vi "GB Test for MANU.vi"(8 "error in":errorcluster, 11 "VISA resource name":refnum<visa-resource-name>) -> (0 "error out":errorcluster, 3 "VISA resource name out":refnum<visa-resource-name>)   [LabVIEW 2011, in "GPT-9000.lvlib"]
uses:
  <instrlib>/GPT-9000/GPT-9000.lvlib
panel:
  in  "GB reference value(m£[)":sgl min=0 max=649.9 format="%.1f"
  in  "GB Test Frequency(Hz)":u8(ring)=1 items=["50", "60"]
  in  "GB Test Time(S)":sgl=2.0 min=0.5 max=999.9 format="%.1f"
  in  "GB LO SET resistance value(m£[)":sgl=0.1 min=0.1 max=649.9 format="%.1f"
  in  "GB HI SET resistance value(m£[)":sgl=650.0 min=0.1 max=650 format="%.1f"
  in  "GB current(A)":sgl=3.0 min=3 max=32 format="%.2f"
  in  "Clear Error(True)":bool=TRUE
  in  "ID Query (True)":bool=TRUE
  out "ID Return String":string
  in  "Start":bool
  in  "Stop":bool
  in  "Test number":u8 max=100
  out "Error Message":string
  out "Error LED":bool
  in  "Test name":string="TEST_NAME"
  out "Time":string
  out "Current":string
  out "Impedance":string
  out "READY":bool
  out "TEST":bool
  out "PASS":bool
  out "FAIL":bool
  out "LED":bool
  out "Ready to Start":bool
  in  "Configure RS232 Baud Rate":u32(ring)=115200 items=["9600"=9600, "19200"=19200, "38400"=38400, "57600"=57600, "115200"=115200]
  # "GB Test for MANU Mode"
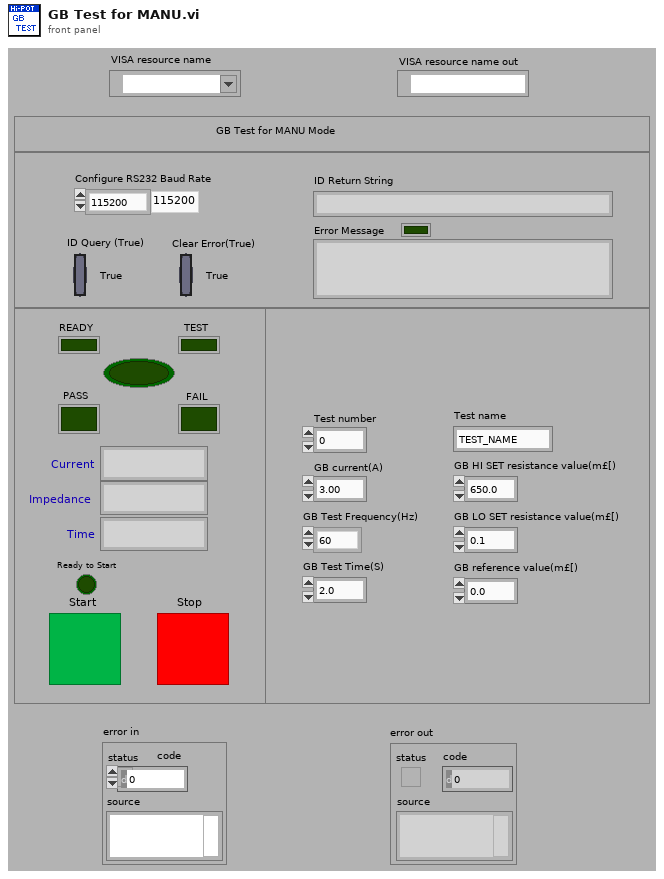
[diagram p1: front panel]
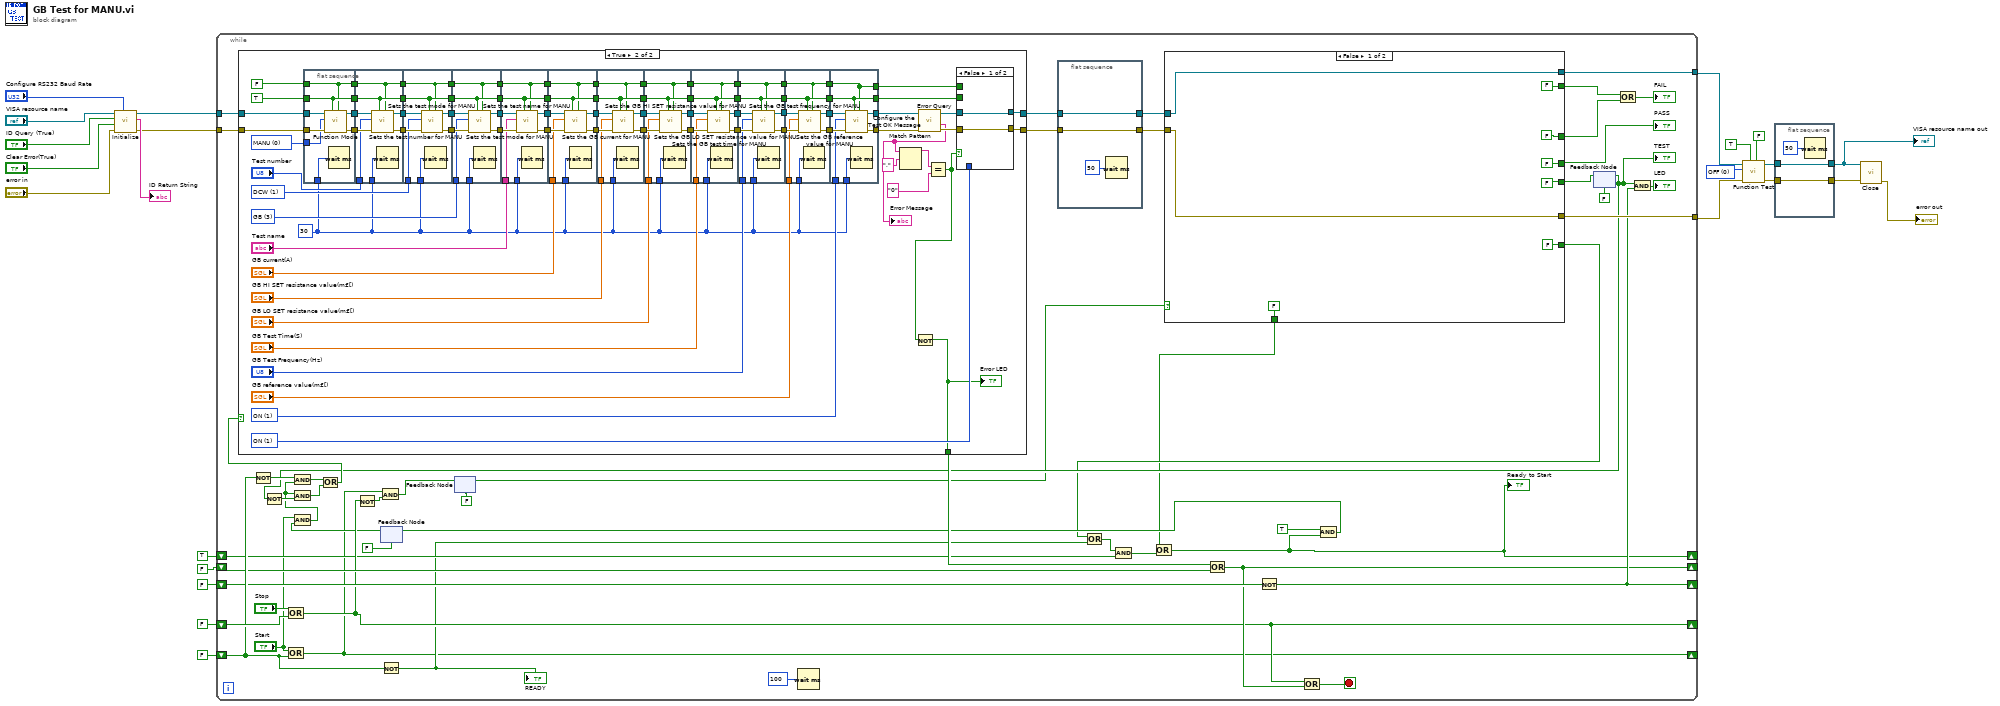
[diagram p0: block diagram]
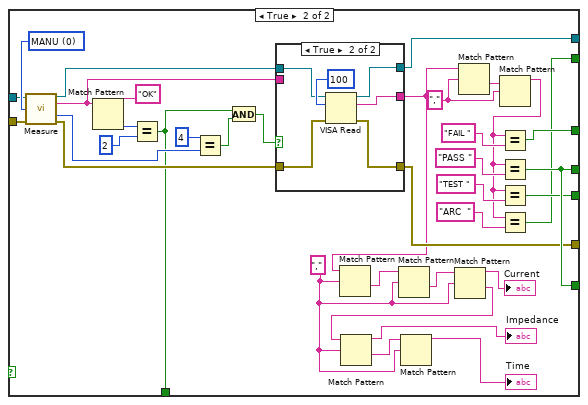
[diagram p2: hidden frame]
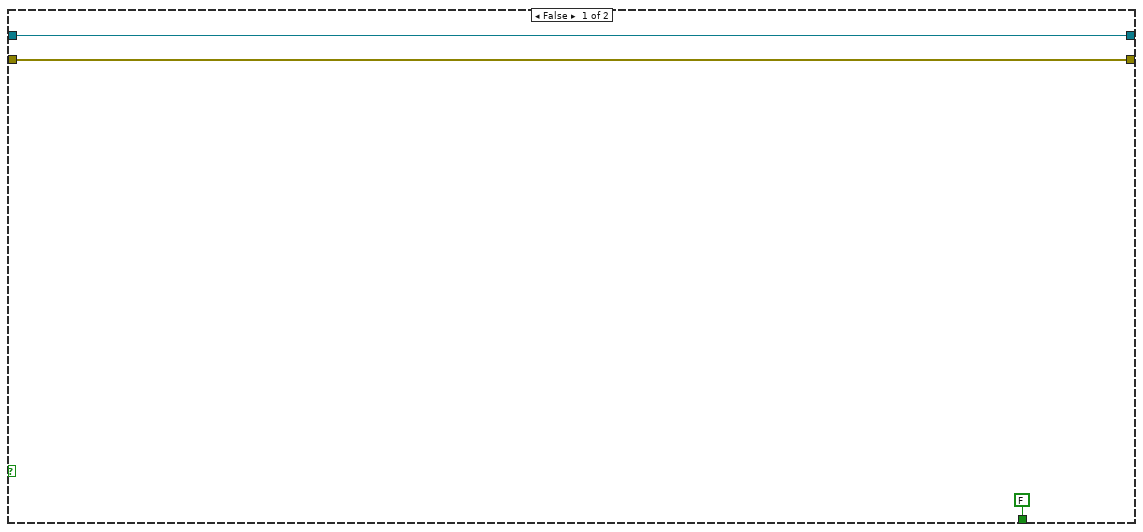
[diagram p4: hidden frame]
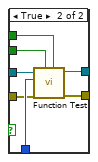
[diagram p5: hidden frame]
diagram:
  w21 = u8 0 items=["OFF", "ON"] ("Function Test")
  n1 = call <instrlib>:"Initialize.vi"("Configure RS232 Baud Rate"="Configure RS232 Baud Rate", "error in (no error)"="error in", "Clear Error(True)"="Clear Error(True)", "ID Query (True)"="ID Query (True)", "VISA resource name"="VISA resource name") -> ("error out"=w10:errorcluster, "ID Return String"=→"ID Return String":string, "VISA resource name out"=w11:refnum<visa-resource-name>)  [unwired: 3 in, 1 out]
  n2 = while {
    shift-right: [w30] -> _
    shift-left: FALSE -> [w66]
    shift-right: [w51] -> _
    shift-left: FALSE -> [w72]
    tunnel: [w71] -> w23
    tunnel: [w70] -> w22
    shift-right: [w65] -> _
    shift-left: FALSE -> [w64]
    tunnel: w11 -> [w58]
    tunnel: w10 -> [w57]
    shift-right: [w54] -> _
    shift-left: FALSE -> [w55]
    shift-right: [w40] -> _
    shift-left: TRUE -> [w45]
    stop <- w56 stop-if-true
    n3 = Not(x=w66) -> (.not. x?=w69:bool)
    n4 = Or(x="Stop", y=w72) -> (x .or. y?=w51:bool)
    n5 = Or(x="Start", y=w66) -> (x .or. y?=w30:bool)
    n6 = Not(x=w51) -> (.not. x?=w68:bool)
    n7 = And(x=w30, y=w68) -> (x .and. y?=w67:bool)
    n8 = feedback #1(FALSE) -> (w38:bool)
    n9 = And(x="Start", y=w38) -> (x .and. y?=w42:bool)
    n10 = And(x=w69, y=w42) -> (x .and. y?=w61:bool)
    n11 = Not(x=w66) -> (.not. x?=w43:bool)
    "READY" <- w43
    n12 = feedback-in #2(w67) -> ()
    n13 = feedback #2(FALSE) -> (w29:bool)
    n14 = Wait (ms)(milliseconds to wait=u32 100) -> ()  [unwired: 1 out]
    n15 = flat-sequence {
      tunnel: w27 -> [w76]
      tunnel: [w76] -> w26
      tunnel: w25 -> [w75]
      tunnel: [w75] -> w24
      frame #0 {
        n16 = Wait (ms)(milliseconds to wait=u32 50) -> ()  [unwired: 1 out]
      }
    }
    n17 = case shown="False" w29 {
      tunnel: [w79 w88] -> w71
      tunnel: [w78 w87] -> w70
      tunnel: [FALSE w106] -> w35
      tunnel: [FALSE w115] -> w32
      tunnel: [FALSE w106] -> w47
      tunnel: [FALSE w105] -> w50
      tunnel: [FALSE w103] -> w31
      tunnel: w26 -> [w79 w90]
      tunnel: w24 -> [w78 w89]
      tunnel: [FALSE w85] -> w28
      frame False {
      }
      frame True {
        w101 = u8 0 items=["MANU", "AUTO"] ("Function Mode Numeric")
        w107 = "," ("regular expression")
        w117 = "," ("regular expression")
        n18 = call <instrlib>:"Measure.vi"("VISA resource name"=w90, "Function Mode Numeric"=w101, "error in"=w89) -> ("VISA resource name out"=w97:refnum<visa-resource-name>, "Return  the test status"=w91:string, "Return the String Count"=w93:u16, "error out"=w96:errorcluster)  [unwired: 9 in]
        n19 = Match Pattern(string=w91, regular expression="OK") -> (offset past match=w99:i32)  [unwired: 1 in, 3 out]
        n20 = Equal?(x=w99, y=2) -> (x = y?=w85:bool)
        n21 = Equal?(x=u16 4, y=w93) -> (x = y?=w94:bool)
        n22 = And(x=w85, y=w94) -> (x .and. y?=w95:bool)
        n23 = case shown="True" w95 {
          tunnel: w96 -> [w123 w124]
          tunnel: [w122 w128] -> w88
          tunnel: [w123 w127] -> w87
          tunnel: [w121 w126] -> w86
          tunnel: w97 -> [w122 w125]
          tunnel: w91 -> [w121 _]
          frame False {
          }
          frame True {
            n24 = VISA Read(VISA resource name=w125, byte count=u32 100, error in (no error)=w124) -> (VISA resource name out=w128:refnum<visa-resource-name>, read buffer=w126:string, error out=w127:errorcluster)  [unwired: 1 out]
          }
        }
        n25 = Match Pattern(string=w86, regular expression=w107) -> (after substring=w114:string)  [unwired: 1 in, 3 out]
        n26 = Match Pattern(string=w114, regular expression=w107) -> (after substring=w110:string)  [unwired: 1 in, 3 out]
        n27 = Match Pattern(string=w110, regular expression=w107) -> (before substring=→"Current":string, after substring=w108:string)  [unwired: 1 in, 2 out]
        n28 = Match Pattern(string=w108, regular expression=w107) -> (before substring=→"Impedance":string, after substring=w113:string)  [unwired: 1 in, 2 out]
        n29 = Match Pattern(string=w113, regular expression=w107) -> (before substring=→"Time":string)  [unwired: 1 in, 3 out]
        n30 = Match Pattern(string=w86, regular expression=w117) -> (after substring=w118:string)  [unwired: 1 in, 3 out]
        n31 = Match Pattern(string=w118, regular expression=w117) -> (before substring=w102:string)  [unwired: 1 in, 3 out]
        n32 = Equal?(x=w102, y="FAIL ") -> (x = y?=w115:bool)
        n33 = Equal?(x=w102, y="PASS ") -> (x = y?=w106:bool)
        n34 = Equal?(x=w102, y="TEST ") -> (x = y?=w105:bool)
        n35 = Equal?(x=w102, y="ARC  ") -> (x = y?=w103:bool)
      }
    }
    "PASS" <- w47
    n36 = Or(x=w35, y=w43) -> (x .or. y?=w44:bool)
    n37 = And(x=w44, y=w45) -> (x .and. y?=w46:bool)
    n38 = Or(x=w28, y=w46) -> (x .or. y?=w40:bool)
    "Ready to Start" <- w40
    n39 = Not(x=w64) -> (.not. x?=w65:bool)
    n40 = And(x=TRUE, y=w40) -> (x .and. y?=w36:bool)
    n41 = feedback-in #1(w36) -> ()
    n42 = feedback-in #3(w50) -> ()
    n43 = feedback #3(FALSE) -> (w49:bool)
    "TEST" <- w49
    n44 = Not(x=w49) -> (.not. x?=w59:bool)
    n45 = And(x=w42, y=w59) -> (x .and. y?=w60:bool)
    n46 = Or(x=w61, y=w60) -> (x .or. y?=w52:bool)
    n47 = case shown="True" w52 {
      tunnel: w58 -> [w132 w197]
      tunnel: w57 -> [w131 w196]
      tunnel: [w132 w205] -> w27
      tunnel: [w131 w204] -> w25
      tunnel: [FALSE w198] -> w53
      frame False {
      }
      frame True {
        w133 = u32 30 ("milliseconds to wait")
        w143 = u8 1 items=["ACW", "DCW", "IR", "GB"] ("Test Mode")
        w134 = u8 1 items=["OFF", "ON"] ("Send Message when test stop")
        w142 = u8 3 items=["ACW", "DCW", "IR", "GB"] ("Test Mode")
        w145 = u8 0 items=["AUTO"=1, "MANU"=0] ("Function Mode")
        w208 = u8 1 items=["OFF", "ON"] ("Function Test")
        n48 = flat-sequence {
          tunnel: w197 -> [w216]
          tunnel: w196 -> [w215]
          tunnel: [w214] -> w195
          tunnel: [w213] -> w194
          tunnel: TRUE -> [w212]
          tunnel: FALSE -> [w211]
          tunnel: [w212] -> w169
          tunnel: [w211] -> w157
          tunnel: w145 -> [w210]
          tunnel: w133 -> [w209]
          tunnel: w195 -> [w224]
          tunnel: w194 -> [w223]
          tunnel: [w222] -> w193
          tunnel: [w221] -> w192
          tunnel: w169 -> [w220]
          tunnel: [w220] -> w168
          tunnel: w157 -> [w219]
          tunnel: [w219] -> w156
          tunnel: "Test number" -> [w218]
          tunnel: w133 -> [w217]
          tunnel: w193 -> [w232]
          tunnel: w192 -> [w231]
          tunnel: [w230] -> w191
          tunnel: [w229] -> w190
          tunnel: w168 -> [w228]
          tunnel: [w228] -> w167
          tunnel: w156 -> [w227]
          tunnel: [w227] -> w155
          tunnel: w143 -> [w226]
          tunnel: w133 -> [w225]
          tunnel: w191 -> [w240]
          tunnel: w190 -> [w239]
          tunnel: [w238] -> w189
          tunnel: [w237] -> w188
          tunnel: w167 -> [w236]
          tunnel: [w236] -> w166
          tunnel: w155 -> [w235]
          tunnel: [w235] -> w154
          tunnel: w142 -> [w234]
          tunnel: w133 -> [w233]
          tunnel: w189 -> [w248]
          tunnel: w188 -> [w247]
          tunnel: [w246] -> w187
          tunnel: [w245] -> w186
          tunnel: w166 -> [w244]
          tunnel: [w244] -> w165
          tunnel: w154 -> [w243]
          tunnel: [w243] -> w153
          tunnel: "Test name" -> [w242]
          tunnel: w133 -> [w241]
          tunnel: w187 -> [w256]
          tunnel: w186 -> [w255]
          tunnel: [w254] -> w185
          tunnel: [w253] -> w184
          tunnel: w165 -> [w252]
          tunnel: [w252] -> w164
          tunnel: w153 -> [w251]
          tunnel: [w251] -> w152
          tunnel: "GB current(A)" -> [w250]
          tunnel: w133 -> [w249]
          tunnel: w185 -> [w264]
          tunnel: w184 -> [w263]
          tunnel: [w262] -> w183
          tunnel: [w261] -> w182
          tunnel: w164 -> [w260]
          tunnel: [w260] -> w163
          tunnel: w152 -> [w259]
          tunnel: [w259] -> w151
          tunnel: "GB HI SET resistance value(m£[)" -> [w258]
          tunnel: w133 -> [w257]
          tunnel: w183 -> [w272]
          tunnel: w182 -> [w271]
          tunnel: [w270] -> w181
          tunnel: [w269] -> w180
          tunnel: w163 -> [w268]
          tunnel: [w268] -> w162
          tunnel: w151 -> [w267]
          tunnel: [w267] -> w150
          tunnel: "GB LO SET resistance value(m£[)" -> [w266]
          tunnel: w133 -> [w265]
          tunnel: w181 -> [w280]
          tunnel: w180 -> [w279]
          tunnel: [w278] -> w179
          tunnel: [w277] -> w178
          tunnel: w162 -> [w276]
          tunnel: [w276] -> w161
          tunnel: w150 -> [w275]
          tunnel: [w275] -> w149
          tunnel: "GB Test Time(S)" -> [w274]
          tunnel: w133 -> [w273]
          tunnel: w179 -> [w288]
          tunnel: w178 -> [w287]
          tunnel: [w286] -> w177
          tunnel: [w285] -> w176
          tunnel: w161 -> [w284]
          tunnel: [w284] -> w160
          tunnel: w149 -> [w283]
          tunnel: [w283] -> w148
          tunnel: "GB Test Frequency(Hz)" -> [w282]
          tunnel: w133 -> [w281]
          tunnel: w177 -> [w296]
          tunnel: w176 -> [w295]
          tunnel: [w294] -> w175
          tunnel: [w293] -> w174
          tunnel: w160 -> [w292]
          tunnel: [w292] -> w159
          tunnel: w148 -> [w291]
          tunnel: [w291] -> w147
          tunnel: "GB reference value(m£[)" -> [w290]
          tunnel: w133 -> [w289]
          tunnel: w175 -> [w304]
          tunnel: w174 -> [w303]
          tunnel: [w302] -> w173
          tunnel: [w301] -> w172
          tunnel: w159 -> [w300]
          tunnel: [w300] -> w158
          tunnel: w147 -> [w299]
          tunnel: [w299] -> w146
          tunnel: w134 -> [w298]
          tunnel: w133 -> [w297]
          frame #0 {
            n49 = call <instrlib>:"Function Mode.vi"("Enable to Query"=w211, "Enable to Setup"=w212, "error in"=w215, "Function Mode"=w210, "VISA resource name"=w216) -> ("error out"=w213:errorcluster, "VISA resource name out"=w214:refnum<visa-resource-name>)  [unwired: 4 in, 1 out]
            n50 = Wait (ms)(milliseconds to wait=w209) -> ()  [unwired: 1 out]
          }
          frame #1 {
            n51 = call <instrlib>:"Sets the test number for MANU.vi"("Enable to Query"=w219, "Enable to Setup"=w220, "error in"=w223, "Test number"=w218, "VISA resource name"=w224) -> ("error out"=w221:errorcluster, "VISA resource name out"=w222:refnum<visa-resource-name>)  [unwired: 4 in, 1 out]
            n52 = Wait (ms)(milliseconds to wait=w217) -> ()  [unwired: 1 out]
          }
          frame #2 {
            n53 = call <instrlib>:"Sets the test mode for MANU.vi"("Enable to Query"=w227, "Enable to Setup"=w228, "error in"=w231, "Test Mode"=w226, "VISA resource name"=w232) -> ("error out"=w229:errorcluster, "VISA resource name out"=w230:refnum<visa-resource-name>)  [unwired: 4 in, 1 out]
            n54 = Wait (ms)(milliseconds to wait=w225) -> ()  [unwired: 1 out]
          }
          frame #3 {
            n55 = call <instrlib>:"Sets the test mode for MANU.vi"("Enable to Query"=w235, "Enable to Setup"=w236, "error in"=w239, "Test Mode"=w234, "VISA resource name"=w240) -> ("error out"=w237:errorcluster, "VISA resource name out"=w238:refnum<visa-resource-name>)  [unwired: 4 in, 1 out]
            n56 = Wait (ms)(milliseconds to wait=w233) -> ()  [unwired: 1 out]
          }
          frame #4 {
            n57 = call <instrlib>:"Sets the test name for MANU.vi"("Enable to Query"=w243, "Enable to Setup"=w244, "error in"=w247, "Test name"=w242, "VISA resource name"=w248) -> ("error out"=w245:errorcluster, "VISA resource name out"=w246:refnum<visa-resource-name>)  [unwired: 4 in, 1 out]
            n58 = Wait (ms)(milliseconds to wait=w241) -> ()  [unwired: 1 out]
          }
          frame #5 {
            n59 = call <instrlib>:"Sets the GB current for MANU.vi"("Enable to Query"=w251, "Enable to Setup"=w252, "error in"=w255, "GB current(A)"=w250, "VISA resource name"=w256) -> ("error out"=w253:errorcluster, "VISA resource name out"=w254:refnum<visa-resource-name>)  [unwired: 4 in, 1 out]
            n60 = Wait (ms)(milliseconds to wait=w249) -> ()  [unwired: 1 out]
          }
          frame #6 {
            n61 = call <instrlib>:"Sets the GB HI SET resistance value for MANU.vi"("Enable to Query"=w259, "Enable to Setup"=w260, "error in"=w263, "GB HI SET resistance value(m£[)"=w258, "VISA resource name"=w264) -> ("error out"=w261:errorcluster, "VISA resource name out"=w262:refnum<visa-resource-name>)  [unwired: 4 in, 1 out]
            n62 = Wait (ms)(milliseconds to wait=w257) -> ()  [unwired: 1 out]
          }
          frame #7 {
            n63 = call <instrlib>:"Sets the GB LO SET resistance value for MANU.vi"("Enable to Query"=w267, "Enable to Setup"=w268, "error in"=w271, "GB LO SET resistance value(m£[)"=w266, "VISA resource name"=w272) -> ("error out"=w269:errorcluster, "VISA resource name out"=w270:refnum<visa-resource-name>)  [unwired: 3 in, 1 out]
            n64 = Wait (ms)(milliseconds to wait=w265) -> ()  [unwired: 1 out]
          }
          frame #8 {
            n65 = call <instrlib>:"Sets the GB test time for MANU.vi"("Enable to Query"=w275, "Enable to Setup"=w276, "error in"=w279, "GB Test Time(S)"=w274, "VISA resource name"=w280) -> ("error out"=w277:errorcluster, "VISA resource name out"=w278:refnum<visa-resource-name>)  [unwired: 4 in, 1 out]
            n66 = Wait (ms)(milliseconds to wait=w273) -> ()  [unwired: 1 out]
          }
          frame #9 {
            n67 = call <instrlib>:"Sets the GB test frequency for MANU.vi"("Enable to Query"=w283, "Enable to Setup"=w284, "error in"=w287, "GB Test Frequency(Hz)"=w282, "VISA resource name"=w288) -> ("error out"=w285:errorcluster, "VISA resource name out"=w286:refnum<visa-resource-name>)  [unwired: 4 in, 1 out]
            n68 = Wait (ms)(milliseconds to wait=w281) -> ()  [unwired: 1 out]
          }
          frame #10 {
            n69 = call <instrlib>:"Sets the GB reference value for MANU.vi"("Enable to Query"=w291, "Enable to Setup"=w292, "error in"=w295, "GB reference value(m£[)"=w290, "VISA resource name"=w296) -> ("error out"=w293:errorcluster, "VISA resource name out"=w294:refnum<visa-resource-name>)  [unwired: 4 in, 1 out]
            n70 = Wait (ms)(milliseconds to wait=w289) -> ()  [unwired: 1 out]
          }
          frame #11 {
            n71 = call <instrlib>:"Configure the Test OK Message.vi"("Query the Message"=w299, "Setup the Message"=w300, "error in"=w303, "Send Message when test stop"=w298, "VISA resource name"=w304) -> ("error out"=w301:errorcluster, "VISA resource name out"=w302:refnum<visa-resource-name>)  [unwired: 4 in, 1 out]
            n72 = Wait (ms)(milliseconds to wait=w297) -> ()  [unwired: 1 out]
          }
        }
        n73 = call <instrlib>:"Error Query.vi"("error in (no error)"=w172, "VISA resource name"=w173) -> ("error out"=w206:errorcluster, "Error Message"=w200:string, "VISA resource name out"=w207:refnum<visa-resource-name>)  [unwired: 6 in, 1 out]
        "Error Message" <- w200
        n74 = Match Pattern(string=w200, regular expression=",") -> (before substring=w202:string)  [unwired: 1 in, 3 out]
        n75 = Equal?(x=w202, y="0") -> (x = y?=w199:bool)
        n76 = Not(x=w199) -> (.not. x?=w198:bool)
        "Error LED" <- w198
        n77 = case shown="False" w199 {
          tunnel: w208 -> [_ w313]
          tunnel: w207 -> [w306 w312]
          tunnel: w206 -> [w305 w311]
          tunnel: [w306 w310] -> w205
          tunnel: [w305 w309] -> w204
          tunnel: w158 -> [_ w308]
          tunnel: w146 -> [_ w307]
          frame False {
          }
          frame True {
            n78 = call <instrlib>:"Function Test.vi"("VISA resource name"=w312, "Function Test"=w313, "error in"=w311, "Enable to Setup"=w308, "Enable to Query"=w307) -> ("VISA resource name out"=w310:refnum<visa-resource-name>, "error out"=w309:errorcluster)  [unwired: 3 in, 1 out]
          }
        }
      }
    }
    n79 = Or(x=w53, y=w55) -> (x .or. y?=w54:bool)
    n80 = Or(x=w51, y=w54) -> (x .or. y?=w56:bool)
    n81 = Or(x=w31, y=w32) -> (x .or. y?=→"FAIL":bool)
    n82 = And(x=w49, y=w65) -> (x .and. y?=→"LED":bool)
  }
  n83 = call <instrlib>:"Function Test.vi"("VISA resource name"=w23, "Function Test"=w21, "error in"=w22, "Enable to Setup"=TRUE, "Enable to Query"=FALSE) -> ("VISA resource name out"=w5:refnum<visa-resource-name>, "error out"=w3:errorcluster)  [unwired: 3 in, 1 out]
  n84 = flat-sequence {
    tunnel: w5 -> [w316]
    tunnel: [w316] -> w4
    tunnel: w3 -> [w315]
    tunnel: [w315] -> w2
    frame #0 {
      n85 = Wait (ms)(milliseconds to wait=u32 50) -> ()  [unwired: 1 out]
    }
  }
  n86 = call <instrlib>:"Close.vi"("error in (no error)"=w2, "VISA resource name"=w4) -> ("error out"=→"error out":errorcluster)  [unwired: 9 in]
  "VISA resource name out" <- w4
